vi "Rubix Cube Array.vi"(7 "Rubix ref Array":refnum<vi>[][](array[refnum]), 8 "error in (no error)":errorcluster, 9 "Rubix Text Array in":string[][](array[string]), 10 "Face to act on":i32, 11 "Command":T2) -> (0 "error out(no error)":errorcluster, 1 "Axis":cluster{"X":sgl, "Y":sgl, "Z":sgl}, 2 "Rubix Array":T1[][](array[typedef]), 3 "Facets To move":T1[](array[typedef]), 5 "Rubix Text Array Out":string[][](array[string]))   [LabVIEW 2019]
uses:
  Cube Data Ops.ctl
  Rubix Array data type.ctl
  Rubix Global data type.ctl
  Rotate array command.ctl
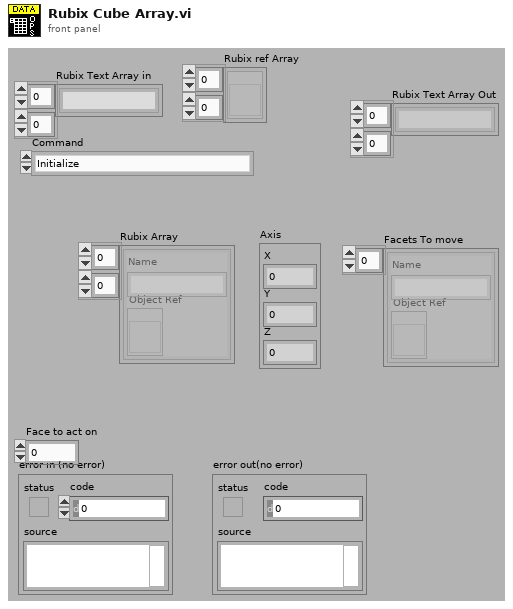
[diagram p1: front panel]
types:
  T1 = typedef "Rubix Array data type.ctl" = cluster{"Object Ref":refnum<vi>, "Name":string}
  T2 = typedef "Cube Data Ops.ctl" = enum16{"Initialize", "Set Rubix Ref Array", "Set Rubix Text Array", "Set Current Face", "Get Rubix Text Array", "Generate Rubix Array", "Get Rubix array", "Get Facets to move", "Randomize", "Top row left", "Top row right", "Middle row left", "Middle row right", "Bottom row left", "Bottom row right", "Left column up", "Left column down", "Middle column up", "Middle column down", "Right column up", "Right column down", "Face ccw", "Face cw"}
  T3 = typedef "Rubix Global data type.ctl" = cluster{"Rubix Text Array":string[][], "Face to act on":i32, "From":i32[], "Axis":cluster{"X":sgl, "Y":sgl, "Z":sgl}, "Rubix ref Array":refnum<vi>[][], "Rubix Array":T1[][], "Facets To move":T1[]}
  T4 = typedef "Rotate array command.ctl" = i32
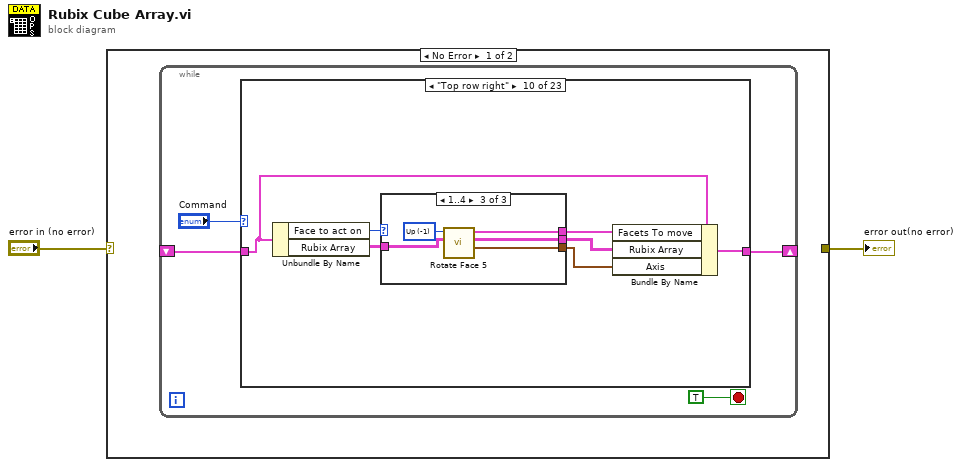
[diagram p0: block diagram]
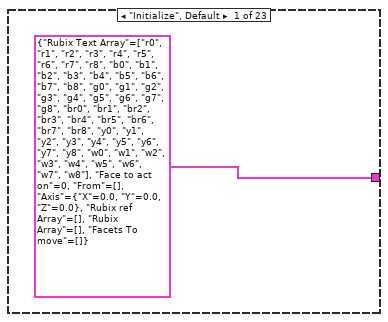
[diagram p2: hidden frame]
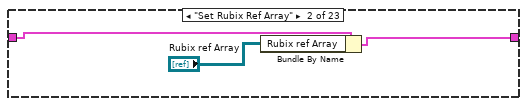
[diagram p3: hidden frame]
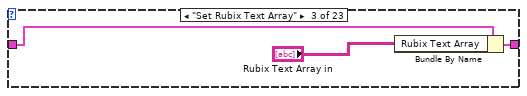
[diagram p4: hidden frame]
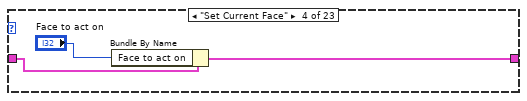
[diagram p5: hidden frame]
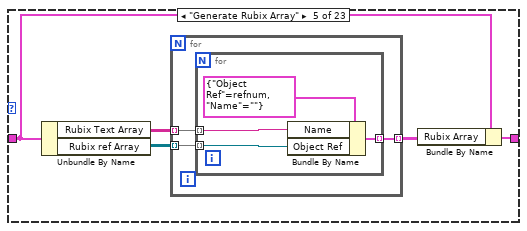
[diagram p6: hidden frame]
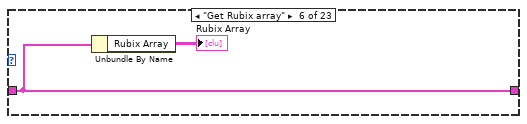
[diagram p7: hidden frame]
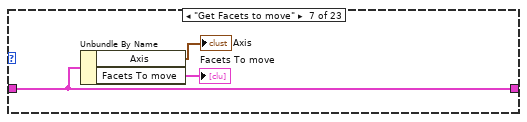
[diagram p8: hidden frame]
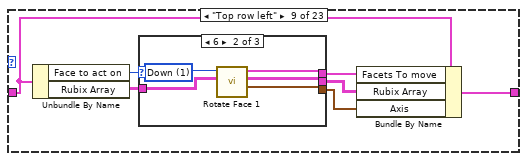
[diagram p10: hidden frame]
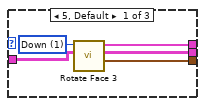
[diagram p11: hidden frame]
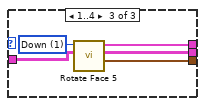
[diagram p12: hidden frame]
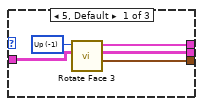
[diagram p13: hidden frame]
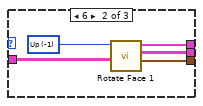
[diagram p14: hidden frame]
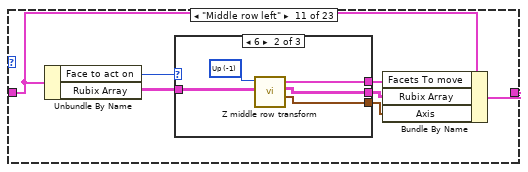
[diagram p15: hidden frame]
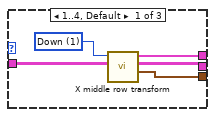
[diagram p16: hidden frame]
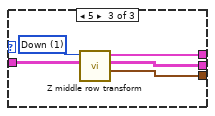
[diagram p17: hidden frame]
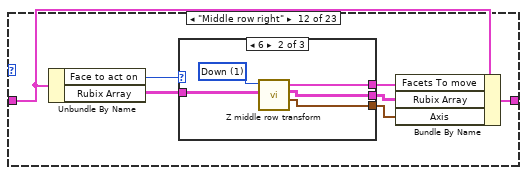
[diagram p18: hidden frame]
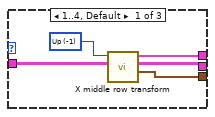
[diagram p19: hidden frame]
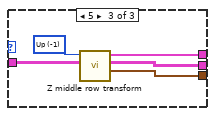
[diagram p20: hidden frame]
diagram:
  n1 = case shown="No Error" "error in (no error)" {
    selector: "error in (no error)" -> [_ w455]
    tunnel: [_ w455] -> w1
    frame No Error {
      n2 = while {
        shift-right: [w4] -> _
        shift-left: _ -> [w3]
        stop <- TRUE stop-if-true
        n3 = case shown="\"Top row right\"" "Command" {
          tunnel: [T3 {"Rubix Text Array"=[["r0", "r1", "r2", "r3", "r4", "r5", "r6", "r7", "r8"], ["b0", "b1", "b2", "b3", "b4", "b5", "b6", "b7", "b8"], ["g0", "g1", "g2", "g3", "g4", "g5", "g6", "g7", "g8"], ["br0", "br1", "br2", "br3", "br4", "br5", "br6", "br7", "br8"], ["y0", "y1", "y2", "y3", "y4", "y5", "y6", "y7", "y8"], ["w0", "w1", "w2", "w3", "w4", "w5", "w6", "w7", "w8"]], "Face to act on"=0, "From"=[], "Axis"={"X"=0.0, "Y"=0.0, "Z"=0.0}, "Rubix ref Array"=[], "Rubix Array"=[], "Facets To move"=[]} ("Cluster") w9 w13 w15 w17 w30 w33 w34 w41 w57 w85 w102 w128 w146 w171 w209 w247 w274 w305 w342 w379 w416 w453] -> w4
          tunnel: w3 -> [_ w10 w11 w16 w19 w30 w33 w34 w35 w58 w84 w101 w127 w145 w172 w208 w241 w273 w306 w343 w380 w417 w453]
          frame "Initialize", Default {
          }
          frame "Set Rubix Ref Array" {
            n4 = Bundle By Name(cluster=w10, "Rubix ref Array"="Rubix ref Array") -> (w9:T3)
          }
          frame "Set Rubix Text Array" {
            n5 = Bundle By Name(cluster=w11, "Rubix Text Array"="Rubix Text Array in") -> (w13:T3)
          }
          frame "Set Current Face" {
            n6 = Bundle By Name(cluster=w16, "Face to act on"="Face to act on") -> (w15:T3)
          }
          frame "Generate Rubix Array" {
            n7 = Unbundle By Name(w19) -> ("Rubix Text Array"=w21:string[][], "Rubix ref Array"=w20:refnum<vi>[][])
            n8 = for {
              tunnel: w21 -> [w24] mode=indexing
              tunnel: w20 -> [w23] mode=indexing
              tunnel: [w22] -> w18 mode=indexing
              n9 = for {
                tunnel: w24 -> [w27] mode=indexing
                tunnel: w23 -> [w25] mode=indexing
                tunnel: [w26] -> w22 mode=indexing
                n10 = Bundle By Name(cluster=T1 {"Object Ref"=refnum, "Name"=""} ("Rubix Array"), "Name"=w27, "Object Ref"=w25) -> (w26:T1)
              }
            }
            n11 = Bundle By Name(cluster=w19, "Rubix Array"=w18) -> (w17:T3)
          }
          frame "Get Rubix array" {
            n12 = Unbundle By Name(w30) -> ("Rubix Array"=→"Rubix Array":T1[][])
          }
          frame "Get Facets to move" {
            n13 = Unbundle By Name(w33) -> ("Axis"=→"Axis":cluster{"X":sgl, "Y":sgl, "Z":sgl}, "Facets To move"=→"Facets To move":T1[])
          }
          frame "Randomize" {
          }
          frame "Top row left" {
            n14 = Unbundle By Name(w35) -> ("Face to act on"=w40:i32, "Rubix Array"=w39:T1[][])
            n15 = case shown="6" w40 {
              tunnel: w39 -> [w43 w47 w55]
              tunnel: [w46 w51 w54] -> w38
              tunnel: [w45 w50 w53] -> w37
              tunnel: [w44 w49 w52] -> w36
              frame 5, Default {
                w42 = T4 1 items=["Up"=-1, "Down"=1] ("Command")
                n16 = call "Rotate Face 3.vi"("Pretransform Rubix Array"=w43, "Command"=w42) -> ("Axis"=w44:cluster{"X":sgl, "Y":sgl, "Z":sgl}, "Transform Rubix Array"=w45:T1[][], "Facets to move"=w46:T1[])  [unwired: 7 in]
              }
              frame 6 {
                w48 = T4 1 items=["Up"=-1, "Down"=1] ("Command")
                n17 = call "Rotate Face 1.vi"("Pretransform Rubix Array"=w47, "Command"=w48) -> ("Axis"=w49:cluster{"X":sgl, "Y":sgl, "Z":sgl}, "Transform Rubix Array"=w50:T1[][], "Facets to move"=w51:T1[])  [unwired: 7 in]
              }
              frame 1..4 {
                w56 = T4 1 items=["Up"=-1, "Down"=1] ("Command")
                n18 = call "Rotate Face 5.vi"("Pretransform Rubix Array"=w55, "Command"=w56) -> ("Axis"=w52:cluster{"X":sgl, "Y":sgl, "Z":sgl}, "Transform Rubix Array"=w53:T1[][], "Facets to move"=w54:T1[])  [unwired: 7 in]
              }
            }
            n19 = Bundle By Name(cluster=w35, "Facets To move"=w38, "Rubix Array"=w37, "Axis"=w36) -> (w41:T3)
          }
          frame "Top row right" {
            n20 = Unbundle By Name(w58) -> ("Face to act on"=w59:i32, "Rubix Array"=w60:T1[][])
            n21 = case shown="1..4" w59 {
              tunnel: w60 -> [w65 w73 w77]
              tunnel: [w68 w71 w76] -> w61
              tunnel: [w67 w70 w75] -> w62
              tunnel: [w66 w69 w74] -> w63
              frame 5, Default {
                w64 = T4 -1 items=["Up"=-1, "Down"=1] ("Command")
                n22 = call "Rotate Face 3.vi"("Pretransform Rubix Array"=w65, "Command"=w64) -> ("Axis"=w66:cluster{"X":sgl, "Y":sgl, "Z":sgl}, "Transform Rubix Array"=w67:T1[][], "Facets to move"=w68:T1[])  [unwired: 7 in]
              }
              frame 6 {
                w72 = T4 -1 items=["Up"=-1, "Down"=1] ("Command")
                n23 = call "Rotate Face 1.vi"("Pretransform Rubix Array"=w73, "Command"=w72) -> ("Axis"=w69:cluster{"X":sgl, "Y":sgl, "Z":sgl}, "Transform Rubix Array"=w70:T1[][], "Facets to move"=w71:T1[])  [unwired: 7 in]
              }
              frame 1..4 {
                w78 = T4 -1 items=["Up"=-1, "Down"=1] ("Command")
                n24 = call "Rotate Face 5.vi"("Pretransform Rubix Array"=w77, "Command"=w78) -> ("Axis"=w74:cluster{"X":sgl, "Y":sgl, "Z":sgl}, "Transform Rubix Array"=w75:T1[][], "Facets to move"=w76:T1[])  [unwired: 7 in]
              }
            }
            n25 = Bundle By Name(cluster=w58, "Facets To move"=w61, "Rubix Array"=w62, "Axis"=w63) -> (w57:T3)
          }
          frame "Middle row left" {
            n26 = Unbundle By Name(w84) -> ("Face to act on"=w83:i32, "Rubix Array"=w79:T1[][])
            n27 = case shown="6" w83 {
              tunnel: [w89 w94 w98] -> w82
              tunnel: [w88 w92 w97] -> w81
              tunnel: [w87 w91 w96] -> w80
              tunnel: w79 -> [w86 w93 w99]
              frame 1..4, Default {
                w90 = T4 1 items=["Up"=-1, "Down"=1] ("Command")
                n28 = call "X middle row transform.vi"("Pretransform Rubix Array"=w86, "Command"=w90) -> ("Axis"=w87:cluster{"X":sgl, "Y":sgl, "Z":sgl}, "Transform Rubix Array"=w88:T1[][], "Facets to move"=w89:T1[])  [unwired: 7 in]
              }
              frame 6 {
                w95 = T4 -1 items=["Up"=-1, "Down"=1] ("Command")
                n29 = call "Z middle row transform.vi"("Pretransform Rubix Array"=w93, "Command"=w95) -> ("Axis"=w91:cluster{"X":sgl, "Y":sgl, "Z":sgl}, "Transform Rubix Array"=w92:T1[][], "Facets to move"=w94:T1[])  [unwired: 7 in]
              }
              frame 5 {
                w100 = T4 1 items=["Up"=-1, "Down"=1] ("Command")
                n30 = call "Z middle row transform.vi"("Pretransform Rubix Array"=w99, "Command"=w100) -> ("Axis"=w96:cluster{"X":sgl, "Y":sgl, "Z":sgl}, "Transform Rubix Array"=w97:T1[][], "Facets to move"=w98:T1[])  [unwired: 7 in]
              }
            }
            n31 = Bundle By Name(cluster=w84, "Facets To move"=w82, "Rubix Array"=w81, "Axis"=w80) -> (w85:T3)
          }
          frame "Middle row right" {
            n32 = Unbundle By Name(w101) -> ("Face to act on"=w103:i32, "Rubix Array"=w107:T1[][])
            n33 = case shown="6" w103 {
              tunnel: [w111 w116 w120] -> w104
              tunnel: [w110 w114 w119] -> w105
              tunnel: [w109 w113 w118] -> w106
              tunnel: w107 -> [w108 w115 w121]
              frame 1..4, Default {
                w112 = T4 -1 items=["Up"=-1, "Down"=1] ("Command")
                n34 = call "X middle row transform.vi"("Pretransform Rubix Array"=w108, "Command"=w112) -> ("Axis"=w109:cluster{"X":sgl, "Y":sgl, "Z":sgl}, "Transform Rubix Array"=w110:T1[][], "Facets to move"=w111:T1[])  [unwired: 7 in]
              }
              frame 6 {
                w117 = T4 1 items=["Up"=-1, "Down"=1] ("Command")
                n35 = call "Z middle row transform.vi"("Pretransform Rubix Array"=w115, "Command"=w117) -> ("Axis"=w113:cluster{"X":sgl, "Y":sgl, "Z":sgl}, "Transform Rubix Array"=w114:T1[][], "Facets to move"=w116:T1[])  [unwired: 7 in]
              }
              frame 5 {
                w122 = T4 -1 items=["Up"=-1, "Down"=1] ("Command")
                n36 = call "Z middle row transform.vi"("Pretransform Rubix Array"=w121, "Command"=w122) -> ("Axis"=w118:cluster{"X":sgl, "Y":sgl, "Z":sgl}, "Transform Rubix Array"=w119:T1[][], "Facets to move"=w120:T1[])  [unwired: 7 in]
              }
            }
            n37 = Bundle By Name(cluster=w101, "Facets To move"=w104, "Rubix Array"=w105, "Axis"=w106) -> (w102:T3)
          }
          frame "Bottom row left" {
            n38 = Unbundle By Name(w127) -> ("Face to act on"=w129:i32, "Rubix Array"=w123:T1[][])
            n39 = case shown="6" w129 {
              tunnel: [w134 w139 w144] -> w126
              tunnel: [w133 w137 w143] -> w125
              tunnel: [w132 w138 w142] -> w124
              tunnel: w123 -> [w131 w135 w140]
              frame 5, Default {
                w130 = T4 -1 items=["Up"=-1, "Down"=1] ("Command")
                n40 = call "Rotate Face 1.vi"("Pretransform Rubix Array"=w131, "Command"=w130) -> ("Axis"=w132:cluster{"X":sgl, "Y":sgl, "Z":sgl}, "Transform Rubix Array"=w133:T1[][], "Facets to move"=w134:T1[])  [unwired: 7 in]
              }
              frame 6 {
                w136 = T4 -1 items=["Up"=-1, "Down"=1] ("Command")
                n41 = call "Rotate Face 3.vi"("Pretransform Rubix Array"=w135, "Command"=w136) -> ("Axis"=w138:cluster{"X":sgl, "Y":sgl, "Z":sgl}, "Transform Rubix Array"=w137:T1[][], "Facets to move"=w139:T1[])  [unwired: 7 in]
              }
              frame 1..4 {
                w141 = T4 1 items=["Up"=-1, "Down"=1] ("Command")
                n42 = call "Rotate Face 6.vi"("Pretransform Rubix Array"=w140, "Command"=w141) -> ("Axis"=w142:cluster{"X":sgl, "Y":sgl, "Z":sgl}, "Transform Rubix Array"=w143:T1[][], "Facets to move"=w144:T1[])  [unwired: 7 in]
              }
            }
            n43 = Bundle By Name(cluster=w127, "Facets To move"=w126, "Rubix Array"=w125, "Axis"=w124) -> (w128:T3)
          }
          frame "Bottom row right" {
            n44 = Unbundle By Name(w145) -> ("Face to act on"=w147:i32, "Rubix Array"=w151:T1[][])
            n45 = case shown="6" w147 {
              tunnel: [w156 w161 w164] -> w148
              tunnel: [w155 w160 w163] -> w149
              tunnel: [w154 w159 w162] -> w150
              tunnel: w151 -> [w153 w158 w165]
              frame 5, Default {
                w152 = T4 1 items=["Up"=-1, "Down"=1] ("Command")
                n46 = call "Rotate Face 1.vi"("Pretransform Rubix Array"=w153, "Command"=w152) -> ("Axis"=w154:cluster{"X":sgl, "Y":sgl, "Z":sgl}, "Transform Rubix Array"=w155:T1[][], "Facets to move"=w156:T1[])  [unwired: 7 in]
              }
              frame 6 {
                w157 = T4 1 items=["Up"=-1, "Down"=1] ("Command")
                n47 = call "Rotate Face 3.vi"("Pretransform Rubix Array"=w158, "Command"=w157) -> ("Axis"=w159:cluster{"X":sgl, "Y":sgl, "Z":sgl}, "Transform Rubix Array"=w160:T1[][], "Facets to move"=w161:T1[])  [unwired: 7 in]
              }
              frame 1..4 {
                w166 = T4 -1 items=["Up"=-1, "Down"=1] ("Command")
                n48 = call "Rotate Face 6.vi"("Pretransform Rubix Array"=w165, "Command"=w166) -> ("Axis"=w162:cluster{"X":sgl, "Y":sgl, "Z":sgl}, "Transform Rubix Array"=w163:T1[][], "Facets to move"=w164:T1[])  [unwired: 7 in]
              }
            }
            n49 = Bundle By Name(cluster=w145, "Facets To move"=w148, "Rubix Array"=w149, "Axis"=w150) -> (w146:T3)
          }
          frame "Left column up" {
            n50 = Unbundle By Name(w172) -> ("Face to act on"=w173:i32, "Rubix Array"=w168:T1[][])
            n51 = case shown="6" w173 {
              tunnel: [w177 w180 w186 w191 w196 w202] -> w170
              tunnel: [w178 w182 w188 w193 w198 w203] -> w167
              tunnel: [w176 w181 w187 w192 w197 w201] -> w169
              tunnel: w168 -> [w175 w179 w185 w190 w195 w200]
              frame 1 {
                w174 = T4 -1 items=["Up"=-1, "Down"=1] ("Command")
                n52 = call "Rotate Face 4.vi"("Pretransform Rubix Array"=w175, "Command"=w174) -> ("Axis"=w176:cluster{"X":sgl, "Y":sgl, "Z":sgl}, "Transform Rubix Array"=w177:T1[][], "Facets to move"=w178:T1[])  [unwired: 7 in]
              }
              frame 2 {
                w183 = T4 -1 items=["Up"=-1, "Down"=1] ("Command")
                n53 = call "Rotate Face 1.vi"("Pretransform Rubix Array"=w179, "Command"=w183) -> ("Axis"=w181:cluster{"X":sgl, "Y":sgl, "Z":sgl}, "Transform Rubix Array"=w180:T1[][], "Facets to move"=w182:T1[])  [unwired: 7 in]
              }
              frame 3 {
                w184 = T4 -1 items=["Up"=-1, "Down"=1] ("Command")
                n54 = call "Rotate Face 2.vi"("Pretransform Rubix Array"=w185, "Command"=w184) -> ("Axis"=w187:cluster{"X":sgl, "Y":sgl, "Z":sgl}, "Transform Rubix Array"=w186:T1[][], "Facets to move"=w188:T1[])  [unwired: 7 in]
              }
              frame 4 {
                w189 = T4 -1 items=["Up"=-1, "Down"=1] ("Command")
                n55 = call "Rotate Face 3.vi"("Pretransform Rubix Array"=w190, "Command"=w189) -> ("Axis"=w192:cluster{"X":sgl, "Y":sgl, "Z":sgl}, "Transform Rubix Array"=w191:T1[][], "Facets to move"=w193:T1[])  [unwired: 7 in]
              }
              frame 5, Default {
                w194 = T4 -1 items=["Up"=-1, "Down"=1] ("Command")
                n56 = call "Rotate Face 4.vi"("Pretransform Rubix Array"=w195, "Command"=w194) -> ("Axis"=w197:cluster{"X":sgl, "Y":sgl, "Z":sgl}, "Transform Rubix Array"=w196:T1[][], "Facets to move"=w198:T1[])  [unwired: 7 in]
              }
              frame 6 {
                w199 = T4 -1 items=["Up"=-1, "Down"=1] ("Command")
                n57 = call "Rotate Face 4.vi"("Pretransform Rubix Array"=w200, "Command"=w199) -> ("Axis"=w201:cluster{"X":sgl, "Y":sgl, "Z":sgl}, "Transform Rubix Array"=w202:T1[][], "Facets to move"=w203:T1[])  [unwired: 7 in]
              }
            }
            n58 = Bundle By Name(cluster=w172, "Facets To move"=w167, "Rubix Array"=w170, "Axis"=w169) -> (w171:T3)
          }
          frame "Left column down" {
            n59 = Unbundle By Name(w208) -> ("Face to act on"=w207:i32, "Rubix Array"=w210:T1[][])
            n60 = case shown="6" w207 {
              tunnel: w210 -> [w211 w217 w222 w229 w232 w237]
              tunnel: [w214 w220 w225 w228 w235 w240] -> w206
              tunnel: [w213 w219 w224 w227 w234 w239] -> w205
              tunnel: [w212 w218 w223 w226 w233 w238] -> w204
              frame 2, Default {
                w215 = T4 1 items=["Up"=-1, "Down"=1] ("Command")
                n61 = call "Rotate Face 1.vi"("Pretransform Rubix Array"=w211, "Command"=w215) -> ("Axis"=w212:cluster{"X":sgl, "Y":sgl, "Z":sgl}, "Transform Rubix Array"=w213:T1[][], "Facets to move"=w214:T1[])  [unwired: 7 in]
              }
              frame 3 {
                w216 = T4 1 items=["Up"=-1, "Down"=1] ("Command")
                n62 = call "Rotate Face 2.vi"("Pretransform Rubix Array"=w217, "Command"=w216) -> ("Axis"=w218:cluster{"X":sgl, "Y":sgl, "Z":sgl}, "Transform Rubix Array"=w219:T1[][], "Facets to move"=w220:T1[])  [unwired: 7 in]
              }
              frame 4 {
                w221 = T4 1 items=["Up"=-1, "Down"=1] ("Command")
                n63 = call "Rotate Face 3.vi"("Pretransform Rubix Array"=w222, "Command"=w221) -> ("Axis"=w223:cluster{"X":sgl, "Y":sgl, "Z":sgl}, "Transform Rubix Array"=w224:T1[][], "Facets to move"=w225:T1[])  [unwired: 7 in]
              }
              frame 5 {
                w230 = T4 1 items=["Up"=-1, "Down"=1] ("Command")
                n64 = call "Rotate Face 4.vi"("Pretransform Rubix Array"=w229, "Command"=w230) -> ("Axis"=w226:cluster{"X":sgl, "Y":sgl, "Z":sgl}, "Transform Rubix Array"=w227:T1[][], "Facets to move"=w228:T1[])  [unwired: 7 in]
              }
              frame 6 {
                w231 = T4 1 items=["Up"=-1, "Down"=1] ("Command")
                n65 = call "Rotate Face 4.vi"("Pretransform Rubix Array"=w232, "Command"=w231) -> ("Axis"=w233:cluster{"X":sgl, "Y":sgl, "Z":sgl}, "Transform Rubix Array"=w234:T1[][], "Facets to move"=w235:T1[])  [unwired: 7 in]
              }
              frame 1 {
                w236 = T4 1 items=["Up"=-1, "Down"=1] ("Command")
                n66 = call "Rotate Face 4.vi"("Pretransform Rubix Array"=w237, "Command"=w236) -> ("Axis"=w238:cluster{"X":sgl, "Y":sgl, "Z":sgl}, "Transform Rubix Array"=w239:T1[][], "Facets to move"=w240:T1[])  [unwired: 7 in]
              }
            }
            n67 = Bundle By Name(cluster=w208, "Facets To move"=w206, "Rubix Array"=w205, "Axis"=w204) -> (w209:T3)
          }
          frame "Middle column up" {
            n68 = Unbundle By Name(w241) -> ("Face to act on"=w246:i32, "Rubix Array"=w245:T1[][])
            n69 = case shown="6" w246 {
              tunnel: w245 -> [w251 w254 w261 w264 w271]
              tunnel: [w250 w256 w259 w266 w269] -> w244
              tunnel: [w249 w257 w260 w267 w270] -> w243
              tunnel: [w248 w255 w258 w265 w268] -> w242
              frame 1, 5 {
                w252 = T4 -1 items=["Up"=-1, "Down"=1] ("Command")
                n70 = call "Y middle colum transform.vi"("Pretransform Rubix Array"=w251, "Command"=w252) -> ("Axis"=w248:cluster{"X":sgl, "Y":sgl, "Z":sgl}, "Transform Rubix Array"=w250:T1[][], "Facets to move"=w249:T1[])  [unwired: 7 in]
              }
              frame 2, Default {
                w253 = T4 1 items=["Up"=-1, "Down"=1] ("Command")
                n71 = call "Z middle row transform.vi"("Pretransform Rubix Array"=w254, "Command"=w253) -> ("Axis"=w255:cluster{"X":sgl, "Y":sgl, "Z":sgl}, "Transform Rubix Array"=w256:T1[][], "Facets to move"=w257:T1[])  [unwired: 7 in]
              }
              frame 3 {
                w262 = T4 1 items=["Up"=-1, "Down"=1] ("Command")
                n72 = call "Y middle colum transform.vi"("Pretransform Rubix Array"=w261, "Command"=w262) -> ("Axis"=w258:cluster{"X":sgl, "Y":sgl, "Z":sgl}, "Transform Rubix Array"=w259:T1[][], "Facets to move"=w260:T1[])  [unwired: 7 in]
              }
              frame 6 {
                w263 = T4 -1 items=["Up"=-1, "Down"=1] ("Command")
                n73 = call "Y middle colum transform.vi"("Pretransform Rubix Array"=w264, "Command"=w263) -> ("Axis"=w265:cluster{"X":sgl, "Y":sgl, "Z":sgl}, "Transform Rubix Array"=w266:T1[][], "Facets to move"=w267:T1[])  [unwired: 7 in]
              }
              frame 4 {
                w272 = T4 -1 items=["Up"=-1, "Down"=1] ("Command")
                n74 = call "Z middle row transform.vi"("Pretransform Rubix Array"=w271, "Command"=w272) -> ("Axis"=w268:cluster{"X":sgl, "Y":sgl, "Z":sgl}, "Transform Rubix Array"=w269:T1[][], "Facets to move"=w270:T1[])  [unwired: 7 in]
              }
            }
            n75 = Bundle By Name(cluster=w241, "Facets To move"=w243, "Rubix Array"=w244, "Axis"=w242) -> (w247:T3)
          }
          frame "Middle column down" {
            n76 = Unbundle By Name(w273) -> ("Face to act on"=w275:i32, "Rubix Array"=w276:T1[][])
            n77 = case shown="4" w275 {
              tunnel: w276 -> [w283 w286 w293 w296 w303]
              tunnel: [w282 w288 w291 w298 w301] -> w277
              tunnel: [w281 w289 w292 w299 w302] -> w278
              tunnel: [w280 w287 w290 w297 w300] -> w279
              frame 1, 5 {
                w284 = T4 1 items=["Up"=-1, "Down"=1] ("Command")
                n78 = call "Y middle colum transform.vi"("Pretransform Rubix Array"=w283, "Command"=w284) -> ("Axis"=w280:cluster{"X":sgl, "Y":sgl, "Z":sgl}, "Transform Rubix Array"=w282:T1[][], "Facets to move"=w281:T1[])  [unwired: 7 in]
              }
              frame 2, Default {
                w285 = T4 -1 items=["Up"=-1, "Down"=1] ("Command")
                n79 = call "Z middle row transform.vi"("Pretransform Rubix Array"=w286, "Command"=w285) -> ("Axis"=w287:cluster{"X":sgl, "Y":sgl, "Z":sgl}, "Transform Rubix Array"=w288:T1[][], "Facets to move"=w289:T1[])  [unwired: 7 in]
              }
              frame 3 {
                w294 = T4 -1 items=["Up"=-1, "Down"=1] ("Command")
                n80 = call "Y middle colum transform.vi"("Pretransform Rubix Array"=w293, "Command"=w294) -> ("Axis"=w290:cluster{"X":sgl, "Y":sgl, "Z":sgl}, "Transform Rubix Array"=w291:T1[][], "Facets to move"=w292:T1[])  [unwired: 7 in]
              }
              frame 6 {
                w295 = T4 1 items=["Up"=-1, "Down"=1] ("Command")
                n81 = call "Y middle colum transform.vi"("Pretransform Rubix Array"=w296, "Command"=w295) -> ("Axis"=w297:cluster{"X":sgl, "Y":sgl, "Z":sgl}, "Transform Rubix Array"=w298:T1[][], "Facets to move"=w299:T1[])  [unwired: 7 in]
              }
              frame 4 {
                w304 = T4 1 items=["Up"=-1, "Down"=1] ("Command")
                n82 = call "Z middle row transform.vi"("Pretransform Rubix Array"=w303, "Command"=w304) -> ("Axis"=w300:cluster{"X":sgl, "Y":sgl, "Z":sgl}, "Transform Rubix Array"=w301:T1[][], "Facets to move"=w302:T1[])  [unwired: 7 in]
              }
            }
            n83 = Bundle By Name(cluster=w273, "Facets To move"=w278, "Rubix Array"=w277, "Axis"=w279) -> (w274:T3)
          }
          frame "Right column up" {
            n84 = Unbundle By Name(w306) -> ("Face to act on"=w307:i32, "Rubix Array"=w310:T1[][])
            n85 = case shown="6" w307 {
              tunnel: [w315 w320 w325 w330 w335 w338] -> w308
              tunnel: [w316 w321 w326 w331 w336 w339] -> w311
              tunnel: [w314 w319 w324 w329 w334 w337] -> w309
              tunnel: w310 -> [w312 w318 w322 w328 w333 w340]
              frame 1 {
                w313 = T4 1 items=["Up"=-1, "Down"=1] ("Command")
                n86 = call "Rotate Face 2.vi"("Pretransform Rubix Array"=w312, "Command"=w313) -> ("Axis"=w314:cluster{"X":sgl, "Y":sgl, "Z":sgl}, "Transform Rubix Array"=w315:T1[][], "Facets to move"=w316:T1[])  [unwired: 7 in]
              }
              frame 2 {
                w317 = T4 1 items=["Up"=-1, "Down"=1] ("Command")
                n87 = call "Rotate Face 3.vi"("Pretransform Rubix Array"=w318, "Command"=w317) -> ("Axis"=w319:cluster{"X":sgl, "Y":sgl, "Z":sgl}, "Transform Rubix Array"=w320:T1[][], "Facets to move"=w321:T1[])  [unwired: 7 in]
              }
              frame 3 {
                w323 = T4 1 items=["Up"=-1, "Down"=1] ("Command")
                n88 = call "Rotate Face 4.vi"("Pretransform Rubix Array"=w322, "Command"=w323) -> ("Axis"=w324:cluster{"X":sgl, "Y":sgl, "Z":sgl}, "Transform Rubix Array"=w325:T1[][], "Facets to move"=w326:T1[])  [unwired: 7 in]
              }
              frame 4 {
                w327 = T4 1 items=["Up"=-1, "Down"=1] ("Command")
                n89 = call "Rotate Face 1.vi"("Pretransform Rubix Array"=w328, "Command"=w327) -> ("Axis"=w329:cluster{"X":sgl, "Y":sgl, "Z":sgl}, "Transform Rubix Array"=w330:T1[][], "Facets to move"=w331:T1[])  [unwired: 7 in]
              }
              frame 5, Default {
                w332 = T4 1 items=["Up"=-1, "Down"=1] ("Command")
                n90 = call "Rotate Face 2.vi"("Pretransform Rubix Array"=w333, "Command"=w332) -> ("Axis"=w334:cluster{"X":sgl, "Y":sgl, "Z":sgl}, "Transform Rubix Array"=w335:T1[][], "Facets to move"=w336:T1[])  [unwired: 7 in]
              }
              frame 6 {
                w341 = T4 1 items=["Up"=-1, "Down"=1] ("Command")
                n91 = call "Rotate Face 2.vi"("Pretransform Rubix Array"=w340, "Command"=w341) -> ("Axis"=w337:cluster{"X":sgl, "Y":sgl, "Z":sgl}, "Transform Rubix Array"=w338:T1[][], "Facets to move"=w339:T1[])  [unwired: 7 in]
              }
            }
            n92 = Bundle By Name(cluster=w306, "Facets To move"=w311, "Rubix Array"=w308, "Axis"=w309) -> (w305:T3)
          }
          frame "Right column down" {
            n93 = Unbundle By Name(w343) -> ("Face to act on"=w348:i32, "Rubix Array"=w345:T1[][])
            n94 = case shown="6" w348 {
              tunnel: [w352 w357 w362 w367 w372 w377] -> w347
              tunnel: [w353 w358 w363 w368 w373 w378] -> w344
              tunnel: [w351 w356 w361 w366 w371 w376] -> w346
              tunnel: w345 -> [w349 w355 w359 w365 w370 w375]
              frame 1 {
                w350 = T4 -1 items=["Up"=-1, "Down"=1] ("Command")
                n95 = call "Rotate Face 2.vi"("Pretransform Rubix Array"=w349, "Command"=w350) -> ("Axis"=w351:cluster{"X":sgl, "Y":sgl, "Z":sgl}, "Transform Rubix Array"=w352:T1[][], "Facets to move"=w353:T1[])  [unwired: 7 in]
              }
              frame 2 {
                w354 = T4 -1 items=["Up"=-1, "Down"=1] ("Command")
                n96 = call "Rotate Face 3.vi"("Pretransform Rubix Array"=w355, "Command"=w354) -> ("Axis"=w356:cluster{"X":sgl, "Y":sgl, "Z":sgl}, "Transform Rubix Array"=w357:T1[][], "Facets to move"=w358:T1[])  [unwired: 7 in]
              }
              frame 3 {
                w360 = T4 -1 items=["Up"=-1, "Down"=1] ("Command")
                n97 = call "Rotate Face 4.vi"("Pretransform Rubix Array"=w359, "Command"=w360) -> ("Axis"=w361:cluster{"X":sgl, "Y":sgl, "Z":sgl}, "Transform Rubix Array"=w362:T1[][], "Facets to move"=w363:T1[])  [unwired: 7 in]
              }
              frame 4 {
                w364 = T4 -1 items=["Up"=-1, "Down"=1] ("Command")
                n98 = call "Rotate Face 1.vi"("Pretransform Rubix Array"=w365, "Command"=w364) -> ("Axis"=w366:cluster{"X":sgl, "Y":sgl, "Z":sgl}, "Transform Rubix Array"=w367:T1[][], "Facets to move"=w368:T1[])  [unwired: 7 in]
              }
              frame 5, Default {
                w369 = T4 -1 items=["Up"=-1, "Down"=1] ("Command")
                n99 = call "Rotate Face 2.vi"("Pretransform Rubix Array"=w370, "Command"=w369) -> ("Axis"=w371:cluster{"X":sgl, "Y":sgl, "Z":sgl}, "Transform Rubix Array"=w372:T1[][], "Facets to move"=w373:T1[])  [unwired: 7 in]
              }
              frame 6 {
                w374 = T4 -1 items=["Up"=-1, "Down"=1] ("Command")
                n100 = call "Rotate Face 2.vi"("Pretransform Rubix Array"=w375, "Command"=w374) -> ("Axis"=w376:cluster{"X":sgl, "Y":sgl, "Z":sgl}, "Transform Rubix Array"=w377:T1[][], "Facets to move"=w378:T1[])  [unwired: 7 in]
              }
            }
            n101 = Bundle By Name(cluster=w343, "Facets To move"=w344, "Rubix Array"=w347, "Axis"=w346) -> (w342:T3)
          }
          frame "Face ccw" {
            n102 = Unbundle By Name(w380) -> ("Face to act on"=w381:i32, "Rubix Array"=w384:T1[][])
            n103 = case shown="1" w381 {
              tunnel: [w389 w394 w399 w404 w409 w414] -> w382
              tunnel: [w390 w395 w400 w405 w410 w415] -> w385
              tunnel: [w388 w393 w398 w403 w408 w413] -> w383
              tunnel: w384 -> [w387 w391 w396 w402 w407 w412]
              frame 1 {
                w386 = T4 -1 items=["Up"=-1, "Down"=1] ("Command")
                n104 = call "Rotate Face 1.vi"("Pretransform Rubix Array"=w387, "Command"=w386) -> ("Axis"=w388:cluster{"X":sgl, "Y":sgl, "Z":sgl}, "Transform Rubix Array"=w389:T1[][], "Facets to move"=w390:T1[])  [unwired: 7 in]
              }
              frame 2 {
                w392 = T4 -1 items=["Up"=-1, "Down"=1] ("Command")
                n105 = call "Rotate Face 2.vi"("Pretransform Rubix Array"=w391, "Command"=w392) -> ("Axis"=w393:cluster{"X":sgl, "Y":sgl, "Z":sgl}, "Transform Rubix Array"=w394:T1[][], "Facets to move"=w395:T1[])  [unwired: 7 in]
              }
              frame 3 {
                w397 = T4 -1 items=["Up"=-1, "Down"=1] ("Command")
                n106 = call "Rotate Face 3.vi"("Pretransform Rubix Array"=w396, "Command"=w397) -> ("Axis"=w398:cluster{"X":sgl, "Y":sgl, "Z":sgl}, "Transform Rubix Array"=w399:T1[][], "Facets to move"=w400:T1[])  [unwired: 7 in]
              }
              frame 4 {
                w401 = T4 -1 items=["Up"=-1, "Down"=1] ("Command")
                n107 = call "Rotate Face 4.vi"("Pretransform Rubix Array"=w402, "Command"=w401) -> ("Axis"=w403:cluster{"X":sgl, "Y":sgl, "Z":sgl}, "Transform Rubix Array"=w404:T1[][], "Facets to move"=w405:T1[])  [unwired: 7 in]
              }
              frame 5, Default {
                w406 = T4 -1 items=["Up"=-1, "Down"=1] ("Command")
                n108 = call "Rotate Face 5.vi"("Pretransform Rubix Array"=w407, "Command"=w406) -> ("Axis"=w408:cluster{"X":sgl, "Y":sgl, "Z":sgl}, "Transform Rubix Array"=w409:T1[][], "Facets to move"=w410:T1[])  [unwired: 7 in]
              }
              frame 6 {
                w411 = T4 1 items=["Up"=-1, "Down"=1] ("Command")
                n109 = call "Rotate Face 6.vi"("Pretransform Rubix Array"=w412, "Command"=w411) -> ("Axis"=w413:cluster{"X":sgl, "Y":sgl, "Z":sgl}, "Transform Rubix Array"=w414:T1[][], "Facets to move"=w415:T1[])  [unwired: 7 in]
              }
            }
            n110 = Bundle By Name(cluster=w380, "Facets To move"=w385, "Rubix Array"=w382, "Axis"=w383) -> (w379:T3)
          }
          frame "Face cw" {
            n111 = Unbundle By Name(w417) -> ("Face to act on"=w422:i32, "Rubix Array"=w419:T1[][])
            n112 = case shown="6" w422 {
              tunnel: [w426 w431 w436 w441 w446 w451] -> w421
              tunnel: [w427 w432 w437 w442 w447 w452] -> w418
              tunnel: [w425 w430 w435 w440 w445 w450] -> w420
              tunnel: w419 -> [w424 w428 w433 w439 w444 w449]
              frame 1 {
                w423 = T4 1 items=["Up"=-1, "Down"=1] ("Command")
                n113 = call "Rotate Face 1.vi"("Pretransform Rubix Array"=w424, "Command"=w423) -> ("Axis"=w425:cluster{"X":sgl, "Y":sgl, "Z":sgl}, "Transform Rubix Array"=w426:T1[][], "Facets to move"=w427:T1[])  [unwired: 7 in]
              }
              frame 2 {
                w429 = T4 1 items=["Up"=-1, "Down"=1] ("Command")
                n114 = call "Rotate Face 2.vi"("Pretransform Rubix Array"=w428, "Command"=w429) -> ("Axis"=w430:cluster{"X":sgl, "Y":sgl, "Z":sgl}, "Transform Rubix Array"=w431:T1[][], "Facets to move"=w432:T1[])  [unwired: 7 in]
              }
              frame 3 {
                w434 = T4 1 items=["Up"=-1, "Down"=1] ("Command")
                n115 = call "Rotate Face 3.vi"("Pretransform Rubix Array"=w433, "Command"=w434) -> ("Axis"=w435:cluster{"X":sgl, "Y":sgl, "Z":sgl}, "Transform Rubix Array"=w436:T1[][], "Facets to move"=w437:T1[])  [unwired: 7 in]
              }
              frame 4 {
                w438 = T4 1 items=["Up"=-1, "Down"=1] ("Command")
                n116 = call "Rotate Face 4.vi"("Pretransform Rubix Array"=w439, "Command"=w438) -> ("Axis"=w440:cluster{"X":sgl, "Y":sgl, "Z":sgl}, "Transform Rubix Array"=w441:T1[][], "Facets to move"=w442:T1[])  [unwired: 7 in]
              }
              frame 5, Default {
                w443 = T4 1 items=["Up"=-1, "Down"=1] ("Command")
                n117 = call "Rotate Face 5.vi"("Pretransform Rubix Array"=w444, "Command"=w443) -> ("Axis"=w445:cluster{"X":sgl, "Y":sgl, "Z":sgl}, "Transform Rubix Array"=w446:T1[][], "Facets to move"=w447:T1[])  [unwired: 7 in]
              }
              frame 6 {
                w448 = T4 -1 items=["Up"=-1, "Down"=1] ("Command")
                n118 = call "Rotate Face 6.vi"("Pretransform Rubix Array"=w449, "Command"=w448) -> ("Axis"=w450:cluster{"X":sgl, "Y":sgl, "Z":sgl}, "Transform Rubix Array"=w451:T1[][], "Facets to move"=w452:T1[])  [unwired: 7 in]
              }
            }
            n119 = Bundle By Name(cluster=w417, "Facets To move"=w418, "Rubix Array"=w421, "Axis"=w420) -> (w416:T3)
          }
          frame "Get Rubix Text Array" {
            n120 = Unbundle By Name(w453) -> ("Rubix Text Array"=→"Rubix Text Array Out":string[][])
          }
        }
      }
    }
    frame Error {
    }
  }
  "error out(no error)" <- w1
